vi "wrap.CreateGLue.vi"(0 "class.GLue in":refnum<class "class.GLue.lvclass">, 7 "Memory":u8[](array[numeric]), 11 "error in (no error)":errorcluster) -> (4 "class.GLue out":refnum<class "class.GLue.lvclass">, 15 "error out":errorcluster)   [LabVIEW 2014, in "GLue.lvlib" / "class.GLue.lvclass"]
uses:
  class.GLue.lvclass
  class.GLue.lvclass/class.GLue.ctl
  Resources/GLue.dll
  Resources/lua52.dll
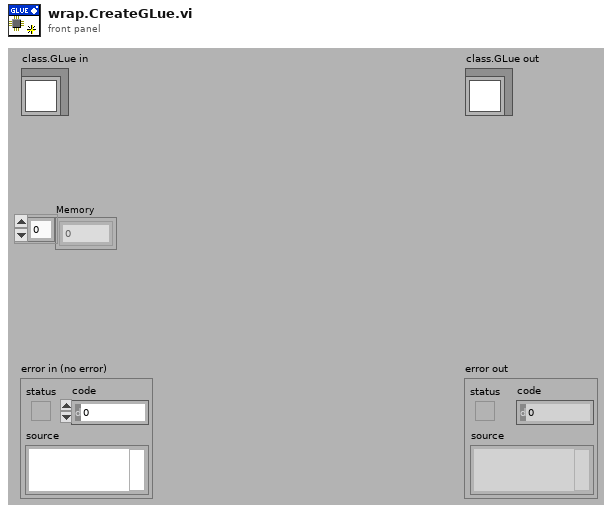
[diagram p1: front panel]
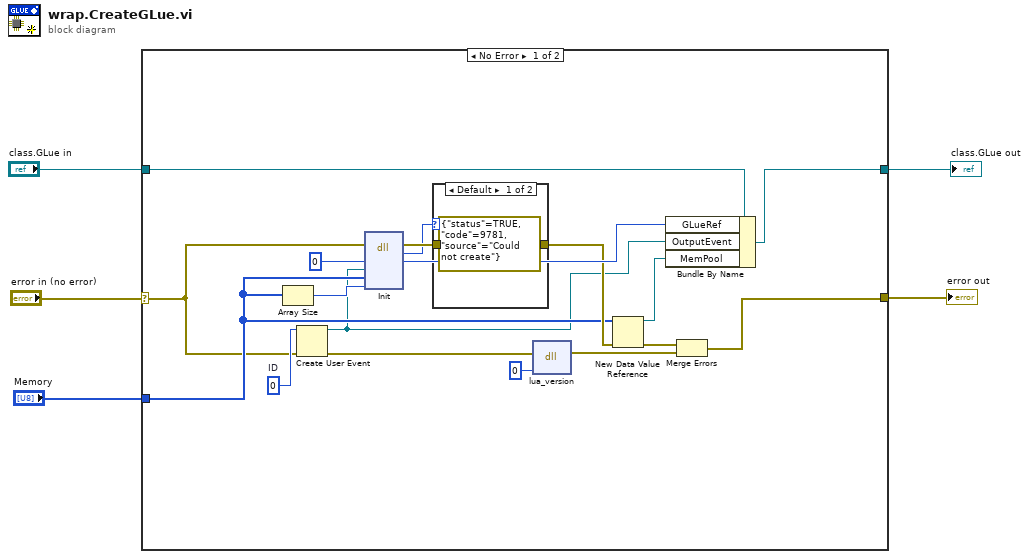
[diagram p0: block diagram]
diagram:
  n1 = case shown="No Error" "error in (no error)" {
    selector: "error in (no error)" -> [w9 w27]
    tunnel: [w21 w27] -> w4
    tunnel: [w22 w26] -> w2
    tunnel: "class.GLue in" -> [w23 w26]
    tunnel: "Memory" -> [w12 _]
    frame No Error {
      w10 = 0  # ID
      n2 = Array Size(array=w12) -> (size(s)=w11:i32)
      n3 = Create User Event(user event datatype=w10, error in=w9) -> (user event=w6:refnum<user-event>, error out=w8:errorcluster)
      n4 = dll-call lib="C:/Users/Antonie/Documents/work/glue/trunk/Resources/GLue.dll" fn="Init"(error in=w9, "GLue"=i64 0 ("MLua"), "outputEvent"=w6, "mempool"=w12, "memsize"=w11) -> (error out=w15:errorcluster, "return type"=w14:i32, "GLue"=w18:i64)  [unwired: 5 in, 1 out]
      n5 = case shown="Default" w14 {
        tunnel: w15 -> [_ w25]
        tunnel: [errorcluster {"status"=TRUE, "code"=9781, "source"="Could not create"} ("error out") w25] -> w13
        frame Default {
        }
        frame 0 {
        }
      }
      n6 = dll-call lib="C:/Users/Antonie/Documents/work/glue/trunk/Resources/lua52.dll" fn="lua_version"(error in=w8, "NULL"=i64 0 ("MLua")) -> (error out=w17:errorcluster)  [unwired: 4 in, 1 out]
      n7 = New Data Value Reference(data value=w12, error in=w13) -> (data value reference=w7:refnum<data-value>, error out=w16:errorcluster)
      n8 = Bundle By Name(cluster=w23, "GLueRef"=w18, "OutputEvent"=w6, "MemPool"=w7) -> (w22:refnum<class "class.GLue.lvclass">)
      n9 = Merge Errors(w16, w17) -> (w21:errorcluster)
    }
    frame Error {
    }
  }
  "error out" <- w4
  "class.GLue out" <- w2
